vi "Pressure Gauge Read.vi"(8 "error in":errorcluster, 10 "task/channels in":refnum<k21>, 11 "Pressure Gauge Type":u16(ring) items=["Dual Mag", "Convectron", "Ion Gauge"]) -> (0 "error out":errorcluster, 3 "element":dbl)   [LabVIEW 2013]
uses:
  <vilib>/DAQmx/read.llb/DAQmx Read.vi
  <vilib>/DAQmx/read.llb/DAQmx Read (Analog 1D DBL NChan 1Samp).vi
  <vilib>/DAQmx/miscellaneous.llb/DAQmx Fill In Error Info.vi
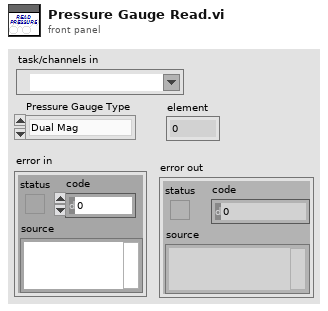
[diagram p1: front panel]
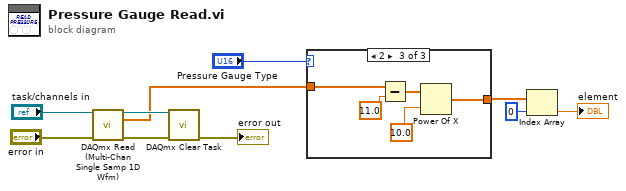
[diagram p0: block diagram]
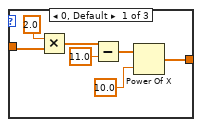
[diagram p2: hidden frame]
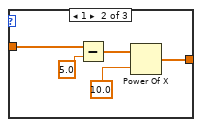
[diagram p3: hidden frame]
diagram:
  n1 = call-poly "DAQmx Read (Multi-Chan Single Samp 1D Wfm).vi"("task/channels in"="task/channels in", "error in"="error in") -> ("task out"=w8:refnum<k21>, "data"=w7:dbl[], "error out"=w9:errorcluster)  [unwired: 11 in]
  n2 = call <vilib>:"DAQmx Clear Task.vi"("task in"=w8, "error in"=w9) -> ("error out"=→"error out":errorcluster)  [unwired: 13 in]
  n3 = case shown="2" "Pressure Gauge Type" {
    tunnel: w7 -> [w14 w21 w25]
    tunnel: [w13 w20 w26] -> w5
    frame 0, Default {
      n4 = Multiply(x=2.0, y=w14) -> (x*y=w16:dbl[])
      n5 = Subtract(x=w16, y=11.0) -> (x-y=w12:dbl[])
      n6 = Power Of X(1:10.0 ("y"), 2:w12) -> (0:w13:dbl[])
    }
    frame 1 {
      n7 = Subtract(x=w21, y=5.0) -> (x-y=w19:dbl[])
      n8 = Power Of X(1:10.0 ("y"), 2:w19) -> (0:w20:dbl[])
    }
    frame 2 {
      n9 = Subtract(x=w25, y=11.0) -> (x-y=w24:dbl[])
      n10 = Power Of X(1:10.0 ("y"), 2:w24) -> (0:w26:dbl[])
    }
  }
  n11 = Index Array(array=w5, index=0) -> (element=→"element":dbl)
